vi "AB_API Is Source Item Present.vi"(8 "error in":errorcluster, 10 "item ID":string, 11 "source items":refnum<class "AB_Source.lvclass">[](array[class])) -> (0 "error out":errorcluster, 2 "index":i32, 3 "source item present?":bool)   [LabVIEW 2020]
uses:
  <vilib>/AppBuilder/AB_Classes/Source/AB_Source.lvclass
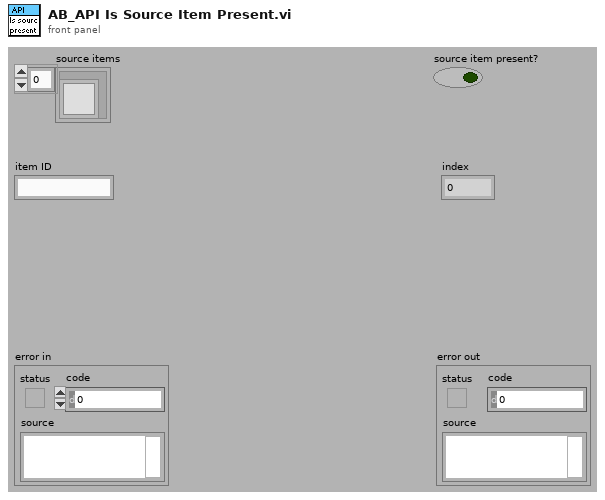
[diagram p1: front panel]
types:
  T1 = typedef "AB_Source.ctl" = cluster{"path":path, "itemID":string, "parentIndex":i32, "sourceInclusion":T2, "destinationIndex":i32, "properties":T3[], "newName":string, "lvfile":bool, "valid":bool, "eng_inBuild":bool, "eng_isNonVILink":bool, "Amalgamation":bool, "Amalgamation Piece":bool, "eng_delimitedName":string, "preventRename":bool}
  T2 = typedef "AB_Source_Inclusion.ctl" = enum16{"IncludeIfReferenced", "Include", "Exclude", "TopLevel"}
  T3 = typedef "AB_Source_Properties.ctl" = cluster{"sourcePropertyType":T4, "value":variant}
  T4 = typedef "AB_Source_Property_Type.ctl" = enum16{"Remove block diagram", "Remove front panel", "Password", "Window has title bar", "Show menu bar", "Show vertical scroll bar", "Show horizontal scroll bar", "Show toolbar", "Show Abort button", "Show fp when called", "Window behavior", "Allow user to close window", "Window run-time position", "Run when opened", "Allow debugging", "Auto error handling", "Generate guard code", "Use stack variables", "Expression folding", "Integer only", "Inline subVI"}
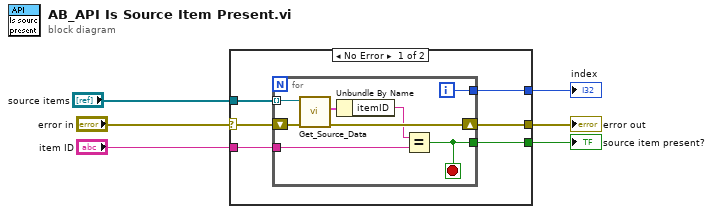
[diagram p0: block diagram]
diagram:
  n1 = case shown="No Error" "error in" {
    selector: "error in" -> [w8 w21]
    tunnel: [w12 _] -> w6
    tunnel: "item ID" -> [w11 _]
    tunnel: [w10 w21] -> w4
    tunnel: "source items" -> [w9 _]
    tunnel: [w7 _] -> w1
    frame No Error {
      n2 = for {
        tunnel: w9 -> [w20] mode=indexing
        shift-right: [w17] -> w10
        shift-left: w8 -> [w18]
        tunnel: w11 -> [w15]
        tunnel: [w14] -> w12
        tunnel: [w13] -> w7
        i -> [w13]
        stop <- w14 stop-if-true
        n3 = call <vilib>:"Get_Source_Data.vi"("error in (no error)"=w18, "Class in"=w20) -> ("error out"=w17:errorcluster, "data"=w19:T1)  [unwired: 8 out]
        n4 = Unbundle By Name(w19) -> ("itemID"=w16:string)
        n5 = Equal?(x=w16, y=w15) -> (x = y?=w14:bool)
      }
    }
    frame Error {
    }
  }
  "source item present?" <- w6
  "error out" <- w4
  "index" <- w1
